vi "Calculate Temperature Change-teardown.vi"(10 "Actual Temperature":dbl, 11 "test case ID":string) -> (3 "result":bool)   [LabVIEW 2018]
doc: "The teardown VI should be executed after the VI under test in the harness VI. In this VI you can evaluate the outputs of the VI under test.\n\nSee the Help Document for more information. (<b>Help</b> > <b>IncQuery Labs</b> > <b>InstaCoverage</b> > <b>InstaCoverage Help...</b>)"
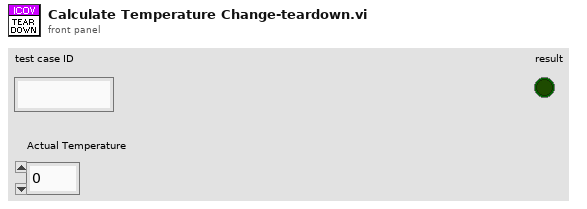
[diagram p1: front panel]
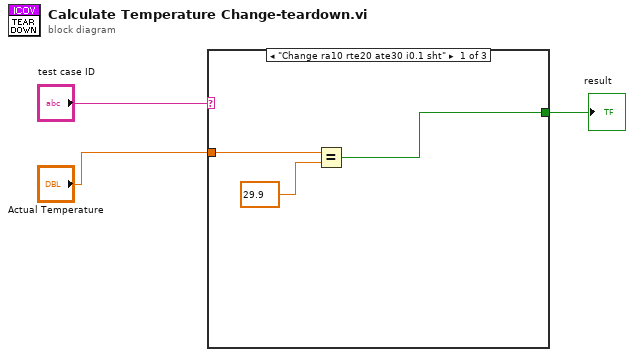
[diagram p0: block diagram]
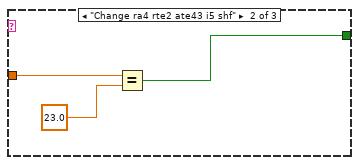
[diagram p2: hidden frame]
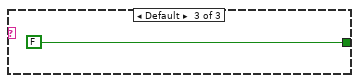
[diagram p3: hidden frame]
diagram:
  n1 = case shown="\"Change ra10 rte20 ate30 i0.1 sht\"" "test case ID" {
    tunnel: [w4 w7 FALSE] -> w2
    tunnel: "Actual Temperature" -> [w5 w8 _]
    frame "Change ra10 rte20 ate30 i0.1 sht" {
      n2 = Equal?(x=w5, y=29.9) -> (x = y?=w4:bool)
    }
    frame "Change ra4 rte2 ate43 i5 shf" {
      n3 = Equal?(x=w8, y=23.0) -> (x = y?=w7:bool)
    }
    frame Default {
    }
  }
  "result" <- w2
